vi "Cleanup.vi"(8 "error in (no error)":errorcluster, 11 "Start Pre-Soak in":refnum<class "Set Desired Station.lvclass">) -> (0 "error out":errorcluster, 3 "Start Pre-Soak out":refnum<class "Set Desired Station.lvclass">)   [LabVIEW 2019, in "Set Desired Station.lvclass"]
uses:
  <vilib>/gpm_packages/@cs/Car-wash/Source/Process Steps/Set Desired Station/Set Desired Station.lvclass
  <vilib>/gpm_packages/@cs/Car-wash/Source/iProcess Step Model/iProcess Step Model/iProcess Step Model.lvclass
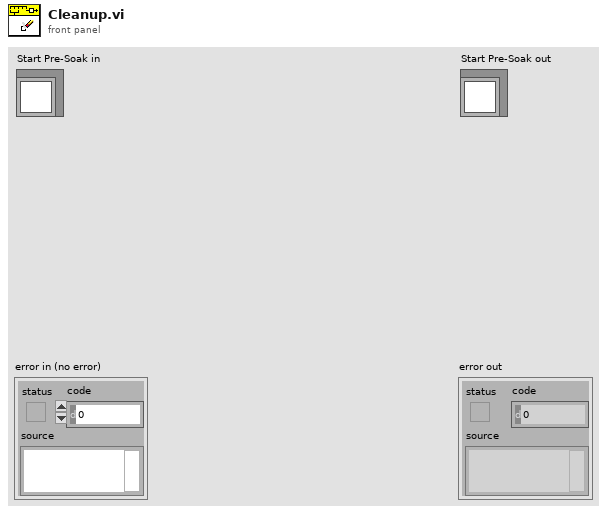
[diagram p1: front panel]
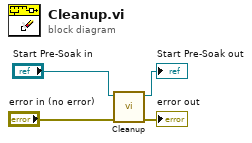
[diagram p0: block diagram]
diagram:
  n1 = call-parent "Cleanup.vi"("error in (no error)"="error in (no error)", "iProcess Step Model in"="Start Pre-Soak in") -> ("error out"=→"error out":errorcluster, "iProcess Step Model out"=→"Start Pre-Soak out":refnum<class "Set Desired Station.lvclass">)  [unwired: 8 in]
